vi "Maintain Heading.vi"(9 "PID gains":T1={"proportional gain (Kc)"=0.02, "integral time (Ti, min)"=0.025, "derivative time (Td, min)"=0.0} {"derivative time (Td, min)" format="%.3f"; "integral time (Ti, min)" format="%.3f"; "proportional gain (Kc)" format="%.3f"}, 10 "NavX Yaw":dbl=-2.8700000000000045, 11 "Raw Driver Joystick X2":dbl) -> (3 "Driver Joystick X2":dbl)   [LabVIEW 2014]
uses:
  <vilib>/Rock Robotics/WPI/DriverStation/WPI_DriverStationRobotMode2.ctl
  Begin/Global Variables.vi
  <vilib>/Utility/file.llb/Write To Spreadsheet File (string).vi
  <vilib>/addons/control/pid/pid.llb/PID (DBL).vi
  <vilib>/addons/control/pid/NI_PID_pid.lvlib
panel:
  in  "Deadband":dbl=0.05 format="%#_13g"
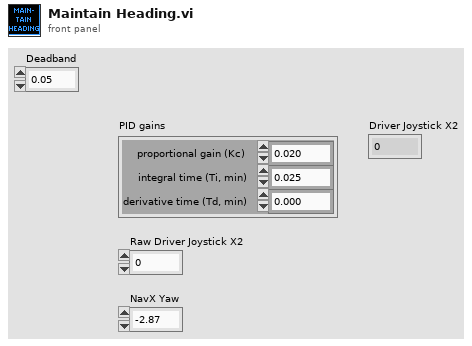
[diagram p1: front panel]
types:
  T1 = cluster{"proportional gain (Kc)":dbl, "integral time (Ti, min)":dbl, "derivative time (Td, min)":dbl}
  T2 = typedef "WPI_DriverStationRobotMode2.ctl" = enum16{"Autonomous Disabled", "Autonomous Enabled", "Teleop Disabled", "Teleop Enabled", "Disconnected", "Finish", "Test Disabled", "Test Enabled", "Emergency Stopped"}
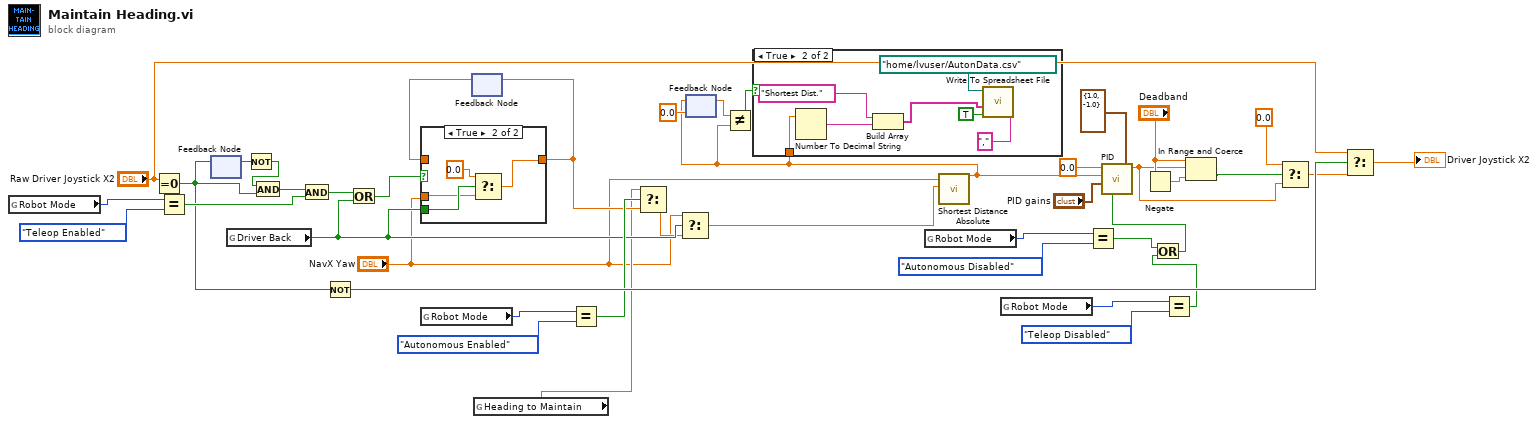
[diagram p0: block diagram]
diagram:
  n1 = global read "Global Variables.vi" "Robot Mode"() -> (w26:T2)
  n2 = Equal To 0?(x="Raw Driver Joystick X2") -> (x = 0?=w29:bool)
  n3 = Equal?(x=w26, y=WPI_DriverStationRobotMode2."Teleop Enabled") -> (x = y?=w40:bool)
  n4 = feedback #1() -> (w31:bool)  [unwired: 1 in]
  n5 = feedback-in #1(w29) -> ()
  n6 = global read "Global Variables.vi" "Driver Back"() -> (w13:bool)
  n7 = Not(x=w31) -> (.not. x?=w30:bool)
  n8 = And(x=w30, y=w29) -> (x .and. y?=w38:bool)
  n9 = And(x=w38, y=w40) -> (x .and. y?=w41:bool)
  n10 = Not(x=w29) -> (.not. x?=w28:bool)
  n11 = Or(x=w41, y=w13) -> (x .or. y?=w42:bool)
  n12 = global read "Global Variables.vi" "Robot Mode"() -> (w23:T2)
  n13 = feedback #2() -> (w27:dbl)  [unwired: 1 in]
  n14 = case shown="True" w42 {
    tunnel: w13 -> [_ w47]
    tunnel: "NavX Yaw" -> [_ w45]
    tunnel: [w43 w44] -> w14
    tunnel: w27 -> [w43 _]
    frame False {
    }
    frame True {
      n15 = Select(t=0.0, s=w47, f=w45) -> (s? t:f=w44:dbl)
    }
  }
  n16 = feedback-in #2(w14) -> ()
  n17 = global read "Global Variables.vi" "Heading to Maintain"() -> (w7:dbl)
  n18 = Equal?(x=w23, y=WPI_DriverStationRobotMode2."Autonomous Enabled") -> (x = y?=w22:bool)
  n19 = Select(t=w7, s=w22, f=w14) -> (s? t:f=w12:dbl)
  n20 = Select(t="NavX Yaw", s=w13, f=w12) -> (s? t:f=w11:dbl)
  n21 = feedback #3(0.0 ("shortest angle")) -> (w4:dbl)
  n22 = global read "Global Variables.vi" "Robot Mode"() -> (w21:T2)
  n23 = call "Shortest Distance Absolute.vi"("current"=w11, "target"="NavX Yaw") -> ("shortest angle"=w1:dbl)  [unwired: 9 in]
  n24 = feedback-in #3(w1) -> ()
  n25 = Not Equal?(x=w4, y=w1) -> (x != y?=w2:bool)
  n26 = case shown="True" w2 {
    tunnel: w1 -> [_ w48]
    frame False {
    }
    frame True {
      n27 = Number To Decimal String(number=w48) -> (decimal integer string=w54:string)  [unwired: 1 in]
      n28 = Build Array("Shortest Dist." ("delimiter (\\t)"), w54) -> (w52:string[])
      n29 = call-poly <vilib>:"Write To Spreadsheet File.vi"("delimiter (\\t)"="," ("delimiter (\\t)"), "append to file? (new file:F)"=TRUE, "1D data"=w52, "file path (dialog if empty)"=path "/home/lvuser/AutonData.csv" ("file path (use dialog)")) -> ()  [unwired: 4 in, 1 out]
    }
  }
  n30 = global read "Global Variables.vi" "Robot Mode"() -> (w18:T2)
  n31 = Equal?(x=w21, y=WPI_DriverStationRobotMode2."Autonomous Disabled") -> (x = y?=w17:bool)
  n32 = Negate(x="Deadband") -> (-x=w37:dbl)
  n33 = Equal?(x=w18, y=WPI_DriverStationRobotMode2."Teleop Disabled") -> (x = y?=w16:bool)
  n34 = Or(x=w17, y=w16) -> (x .or. y?=w15:bool)
  n35 = call-poly <vilib>:"PID.vi"("reinitialize? (F)"=w15, "output range"=cluster{"output high":dbl, "output low":dbl} {"output high"=1.0, "output low"=-1.0}, "PID gains"="PID gains", "process variable"=w1, "setpoint"=0.0) -> ("output"=w9:dbl)  [unwired: 5 in, 1 out]
  n36 = In Range and Coerce(upper limit="Deadband", x=w9, lower limit=w37) -> (In Range?=w10:bool)  [unwired: 1 out]
  n37 = Select(t=0.0, s=w10, f=w9) -> (s? t:f=w8:dbl)
  n38 = Select(t="Raw Driver Joystick X2", s=w28, f=w8) -> (s? t:f=→"Driver Joystick X2":dbl)
